vi "MainProgram.vi"() -> ()   [LabVIEW 2020]
panel:
  out "Position:Left 2":i32
  out "Position:Left":i32
  in  "RE":bool
  in  "Down R":bool
  in  "R-L":bool
  in  "Up":bool
  in  "Hold":bool
  in  "Down":bool
  out "Boolean 2":bool
  out "Boolean":bool
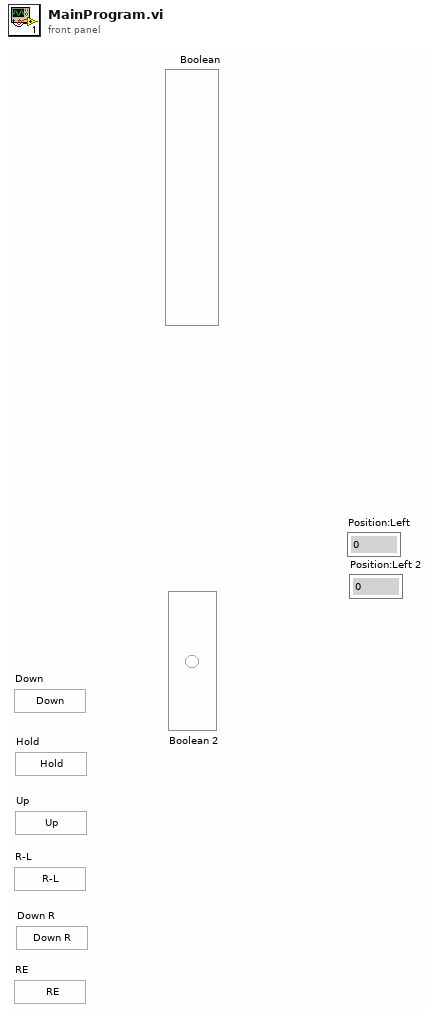
[diagram p1: front panel]
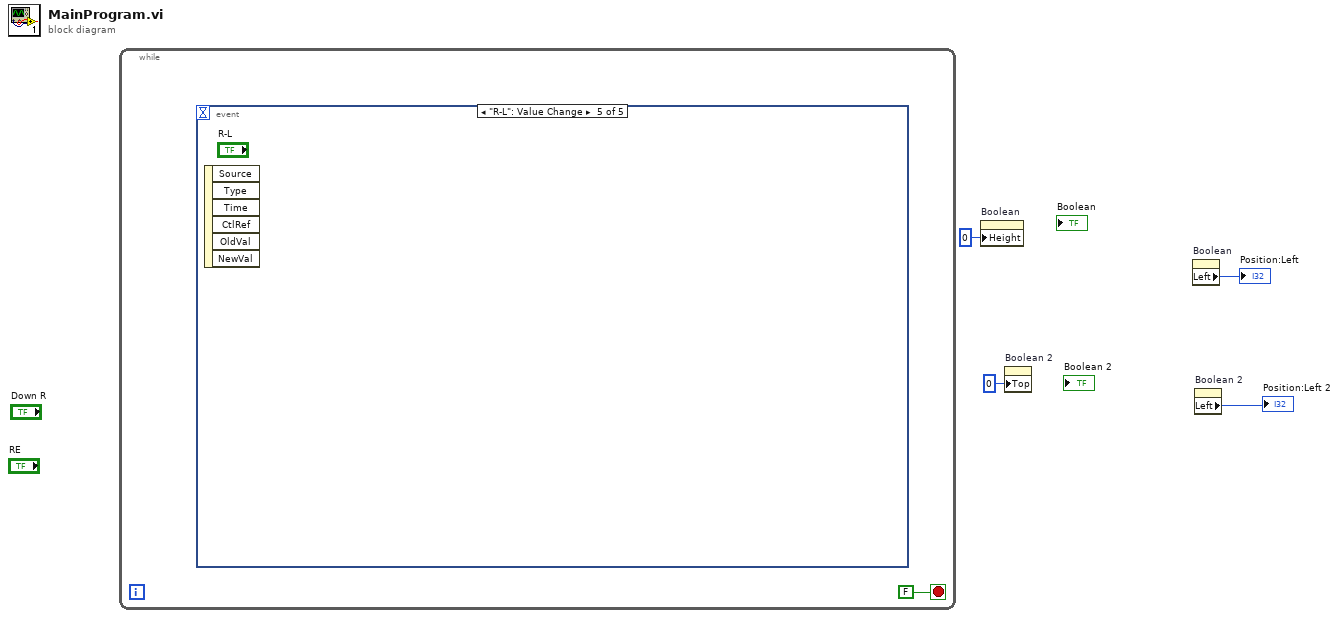
[diagram p0: block diagram]
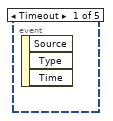
[diagram p2: hidden frame]
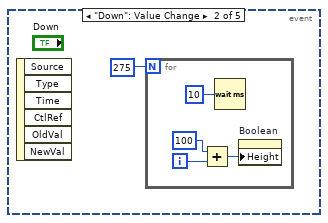
[diagram p3: hidden frame]
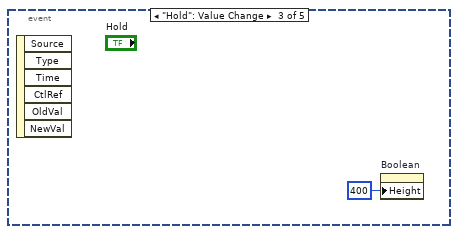
[diagram p4: hidden frame]
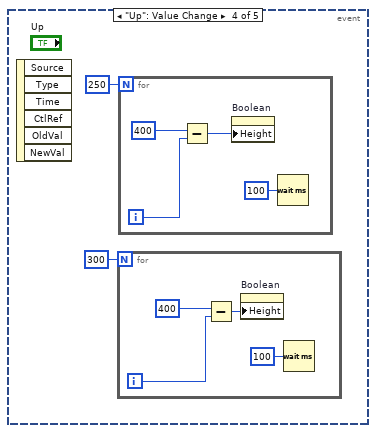
[diagram p5: hidden frame]
diagram:
  n1 = while {
    stop <- FALSE stop-if-true
    n2 = event shown="[4] \"R-L\": Value Change" {
      selector: _ -> [_ _ _ _ _]
      dyn-events: _ -> [_ _ _ _ _]
      timeout: _ -> [_ _ _ _ _]
      event Timeout {
        n3 = event-data() -> ()  [unwired: 1 in, 3 out]
      }
      event "Down": Value Change {
        n4 = event-data() -> ()  [unwired: 1 in, 6 out]
        n5 = for {
          N: 275 -> [_]
          i -> [w7]
          n6 = Add(x=100, y=w7) -> (x+y=w9:i32)
          n7 = Wait (ms)(milliseconds to wait=u32 10) -> ()  [unwired: 1 out]
          n8 = property on="Boolean" class="Bool (strict)"("Height"=w9) -> ()  [unwired: 2 in, 2 out]
        }
      }
      event "Hold": Value Change {
        n9 = event-data() -> ()  [unwired: 1 in, 6 out]
        n10 = property on="Boolean" class="Bool (strict)"("Height"=u32 400 ("Button Size:Height")) -> ()  [unwired: 2 in, 2 out]
      }
      event "Up": Value Change {
        n11 = event-data() -> ()  [unwired: 1 in, 6 out]
        n12 = for {
          N: 300 -> [_]
          i -> [w15]
          n13 = Subtract(x=400, y=w15) -> (x-y=w16:i32)
          n14 = property on="Boolean" class="Bool (strict)"("Height"=w16) -> ()  [unwired: 2 in, 2 out]
          n15 = Wait (ms)(milliseconds to wait=u32 100) -> ()  [unwired: 1 out]
        }
        n16 = for {
          N: 250 -> [_]
          i -> [w20]
          n17 = Subtract(x=400, y=w20) -> (x-y=w19:i32)
          n18 = property on="Boolean" class="Bool (strict)"("Height"=w19) -> ()  [unwired: 2 in, 2 out]
          n19 = Wait (ms)(milliseconds to wait=u32 100) -> ()  [unwired: 1 out]
        }
      }
      event "R-L": Value Change {
        n20 = event-data() -> ()  [unwired: 1 in, 6 out]
      }
    }
  }
  n21 = property on="Boolean" class="Bool (strict)"("Height"=u32 0 ("Button Size:Height")) -> ()  [unwired: 2 in, 2 out]
  n22 = property on="Boolean 2" class="Bool (strict)"("Top"=0 ("Position:Top")) -> ()  [unwired: 2 in, 2 out]
  n23 = property on="Boolean" class="Bool (strict)"() -> ("Left"=→"Position:Left":i32)  [unwired: 2 in, 2 out]
  n24 = property on="Boolean 2" class="Bool (strict)"() -> ("Left"=→"Position:Left 2":i32)  [unwired: 2 in, 2 out]
